vi "Build GOOP Levels.vi"(11 "LabVIEW Object in":refnum<class>) -> (0 "Not a GOOP obj?":bool, 1 "Not a Ref Yet?":bool, 2 "Level's Data (Child -> Parent)":T1[](array[typedef]), 3 "Hash":string)   [LabVIEW 2019, in "GOOP Probe.lvlib"]
uses:
  GOOP Probe.lvlib
  Class intergrator/Class Integrator.lvlib
  Level Data.ctl
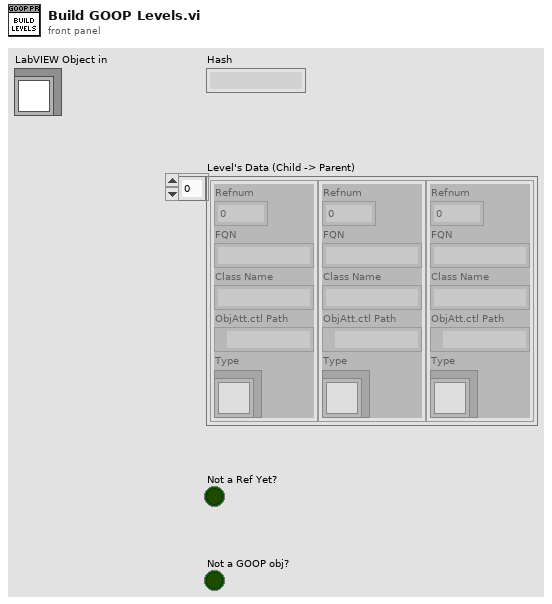
[diagram p1: front panel]
types:
  T1 = typedef "GOOP Probe.lvlib/Level Data.ctl" = cluster{"Refnum":i32, "FQN":string, "Class Name":string, "ObjAtt.ctl Path":path, "Type":refnum<class>}
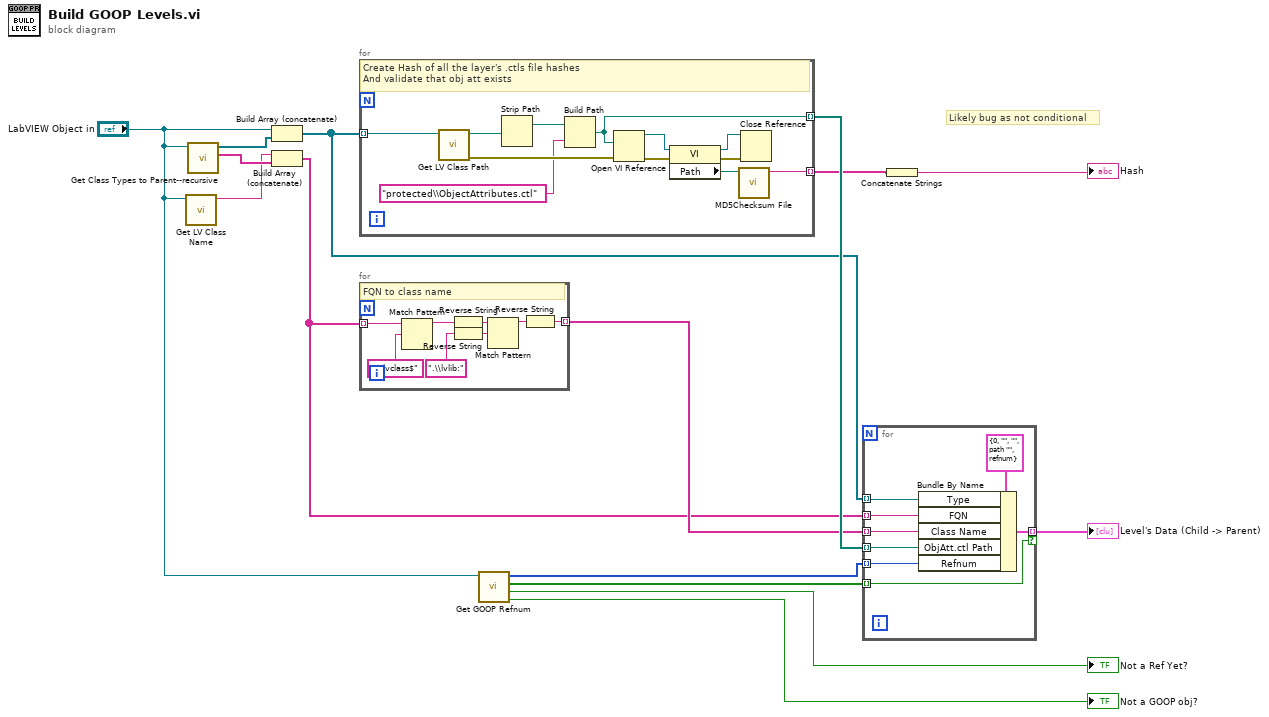
[diagram p0: block diagram]
diagram:
  # "Likely bug as not conditional"
  n1 = call <vilib>:"Get LV Class Name.vi"("object"="LabVIEW Object in") -> ("class name"=w7:string)  [unwired: 9 in, 1 out]
  n2 = call "Get Class Types to Parent--recursive.vi"("Instance"="LabVIEW Object in") -> ("Class Levels To Requested (FQN)"=w8:string[], "Class Levels To Requested (Types)"=w10:refnum<class>[])  [unwired: 8 in, 1 out]
  n3 = Build Array (concatenate)("LabVIEW Object in", w10) -> (w12:refnum<class>[])
  n4 = Build Array (concatenate)(w7, w8) -> (w11:string[])
  n5 = for {
    tunnel: [w16] -> w4 mode=indexing
    tunnel: w12 -> [w19] mode=indexing
    tunnel: [w18] -> w15 mode=indexing
    # "Create Hash of all the layer's .ctls file hashes\nAnd validate that obj att exists"
    n6 = call <vilib>:"Get LV Class Path.vi"("object"=w19) -> ("error out"=w22:errorcluster, "class path"=w23:path)  [unwired: 9 in]
    n7 = Strip Path(path=w23) -> (stripped path=w20:path)  [unwired: 1 out]
    n8 = Build Path(base path=w20, name or relative path="protected\\ObjectAttributes.ctl" ("string")) -> (appended path=w18:path)
    n9 = Open VI Reference(vi path=w18, error in (no error)=w22) -> (vi reference=w27:refnum<vi>, error out=w26:errorcluster)  [unwired: 4 in]
    n10 = property class="VI"(reference=w27, error in=w26) -> (reference out=w24:refnum<vi>, error out=w25:errorcluster, "Path"=w17:path)
    n11 = call <vilib>:"MD5Checksum File.vi"("Path"=w17) -> ("MD5 message-digest"=w16:string)  [unwired: 9 in, 1 out]
    n12 = Close Reference(reference=w24, error in (no error)=w25) -> ()  [unwired: 1 out]
  }
  n13 = for {
    tunnel: w11 -> [w29] mode=indexing
    tunnel: [w28] -> w14 mode=indexing
    # "FQN to class name"
    n14 = Match Pattern(string=w29, regular expression="\\.lvclass$") -> (before substring=w30:string)  [unwired: 1 in, 3 out]
    n15 = Reverse String(1:w30) -> (0:w34:string)
    n16 = Reverse String(1:".\\lvlib:" ("regular expression")) -> (0:w33:string)
    n17 = Match Pattern(string=w34, regular expression=w33) -> (before substring=w32:string)  [unwired: 1 in, 3 out]
    n18 = Reverse String(1:w32) -> (0:w28:string)
  }
  n19 = call "Get GOOP Refnum.vi"("LabVIEW Object in"="LabVIEW Object in") -> ("No Levels a GOOP obj"=→"Not a GOOP obj?":bool, "Not a Ref Yet?"=→"Not a Ref Yet?":bool, "Not Goop by Level"=w5:bool[], "Refnum?"=w13:u32[])  [unwired: 7 in]
  n20 = for {
    tunnel: w13 -> [w42] mode=indexing
    tunnel: w11 -> [w41] mode=indexing
    tunnel: w14 -> [w40] mode=indexing
    tunnel: w15 -> [w39] mode=indexing
    tunnel: [w38] -> w6 mode=indexing if=w36
    tunnel: w5 -> [w36] mode=indexing
    tunnel: w12 -> [w37] mode=indexing
    n21 = Bundle By Name(cluster=T1 {"Refnum"=0, "FQN"="", "Class Name"="", "ObjAtt.ctl Path"=path "", "Type"=refnum}, "Type"=w37, "FQN"=w41, "Class Name"=w40, "ObjAtt.ctl Path"=w39, "Refnum"=w42) -> (w38:T1)
  }
  "Level's Data (Child -> Parent)" <- w6
  n22 = Concatenate Strings(w4) -> (→"Hash":string)
